vi "Update time delay graph.vi"(8 "error in (no error)":errorcluster caption="entrée d'erreur (pas d'erreur)", 11 "Control-Client en entrée":refnum<class "Control-Client.lvclass">) -> (0 "error out":errorcluster caption="sortie d'erreur", 3 "Control-Client en sortie":refnum<class "Control-Client.lvclass">)   [LabVIEW 2018, in "Control-Client.lvclass"]
uses:
  Control-Client.lvclass
  Control-Client.lvclass/Control-Client.ctl
  Experiments/Experiment.lvclass
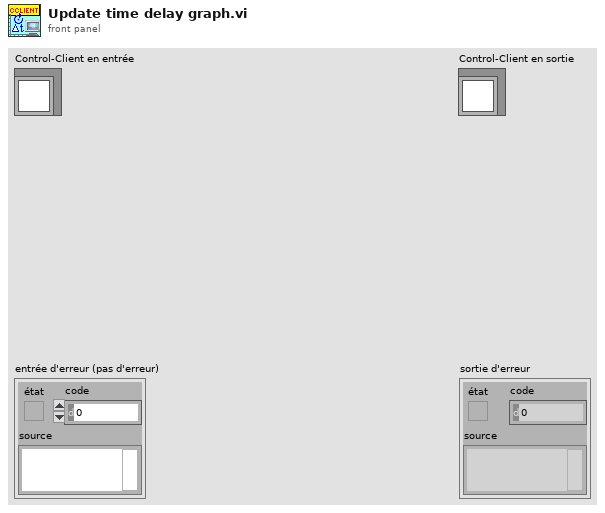
[diagram p1: front panel]
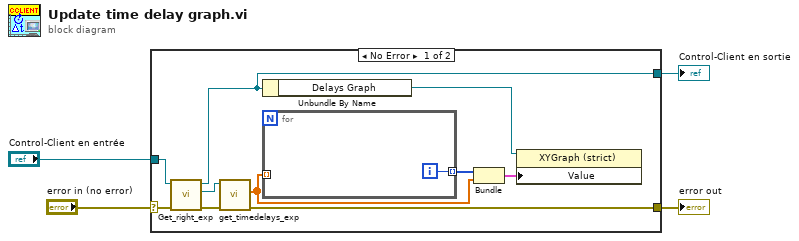
[diagram p0: block diagram]
diagram:
  n1 = case shown="No Error" "error in (no error)" {
    selector: "error in (no error)" -> [w6 w17]
    tunnel: [w10 w17] -> w3
    tunnel: [w8 w16] -> w1
    tunnel: "Control-Client en entrée" -> [w7 w16]
    frame No Error {
      n2 = call "Get_right_exp.vi"("error in (no error)"=w6, "Control-Client in"=w7) -> ("error out"=w5:errorcluster, "Right experiment"=w9:refnum<class "Experiment.lvclass">, "Control-Client out"=w8:refnum<class "Control-Client.lvclass">)  [unwired: 7 in]
      n3 = call "get_timedelays_exp.vi"("error in (no error)"=w5, "Experiment.lvclass in"=w9) -> ("error out"=w10:errorcluster, "timedelays"=w11:dbl[])  [unwired: 7 in, 1 out]
      n4 = Unbundle By Name(w8) -> ("Delays Graph"=w12:refnum<vi>)
      n5 = for {
        tunnel: [w15] -> w13 mode=indexing
        tunnel: w11 -> [_] mode=indexing
        i -> [w15]
      }
      n6 = Bundle(w13, "timedelays"=w11) -> (w14:cluster{i32[], "timedelays":dbl[]})  [unwired: 1 in]
      n7 = property class="XYGraph (strict)"(reference=w12, "Value"=w14) -> ()  [unwired: 1 in, 2 out]
    }
    frame Error {
    }
  }
  "error out" <- w3
  "Control-Client en sortie" <- w1
